vi "GetSupplyVolts.vi"(3 "error in (no error)":errorcluster) -> (0 "error out":errorcluster, 1 "String_Volts":string, 4 "Volts +15":dbl format="%#.10g", 5 "Volts +24":dbl format="%#.10g")   [LabVIEW 2009]
doc: "Read multiple power supply voltages."
panel:
  in  "Volts Spare2":dbl=-999.0 format="%#.10g"
  in  "Volts Spare1":dbl=-999.0 format="%#.10g"
  in  "SCPI command":string="sens:volt:dc:nplc 2,(@1039:1040)\nconf:volt:dc 100,0.0001,(@1039:1040)\nrout:scan (@1039:1040)\ninit\n"
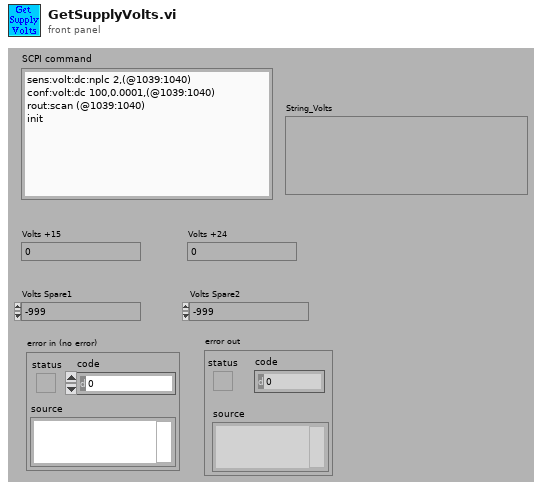
[diagram p1: front panel]
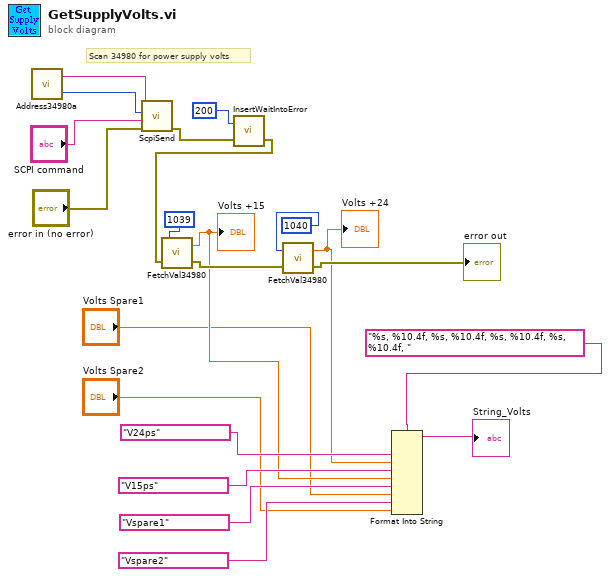
[diagram p0: block diagram]
diagram:
  # "Scan 34980 for power supply volts"
  n1 = call "Address34980a.vi"() -> ("Port"=w18:i32, "IP address"=w19:string)  [unwired: 2 in]
  n2 = call "ScpiSend.vi"("error in (no error)"="error in (no error)", "Command"="SCPI command", "TCP port"=w18, "IP Address"=w19) -> ("error out"=w15:errorcluster)  [unwired: 7 in]
  n3 = call "InsertWaitIntoError.vi"("error in (no error)"=w15, "Wait (msecs)"=200) -> ("error out"=w14:errorcluster)  [unwired: 1 in]
  n4 = call "FetchVal34980.vi"("error in (no error)"=w14, "Circuit ID"=1039) -> ("Error out"=w12:errorcluster, "Value"=w4:dbl)
  "Volts +15" <- w4
  n5 = call "FetchVal34980.vi"("error in (no error)"=w12, "Circuit ID"=1040) -> ("Error out"=→"error out":errorcluster, "Value"=w3:dbl)
  "Volts +24" <- w3
  n6 = Format Into String(format string="%s, %10.4f, %s, %10.4f, %s, %10.4f, %s, %10.4f, ", "V24ps", w3, "V15ps", w4, "Vspare1", "Volts Spare1", "Vspare2", "Volts Spare2") -> (resulting string=→"String_Volts":string)  [unwired: 2 in, 1 out]
